vi "checkFinishPreparePassPlay.vi"(8 "error in (no error)":errorcluster, 10 "Game":refnum<class "Game.lvclass">, 11 "PreparePassPlay in":refnum<class "PreparePassPlay.lvclass">) -> (0 "error out":errorcluster, 2 "Boolean":bool, 3 "PreparePassPlay out":refnum<class "PreparePassPlay.lvclass">)   [LabVIEW 2018, in "PreparePassPlay.lvclass"]
uses:
  PreparePassPlay.lvclass
  Game_class/Game.lvclass
  Game_class/Game.lvclass/Game.ctl
  Referee_class/Referee.lvclass/Referee.ctl
  Events_class/Events.lvclass/Events.ctl
  Team_class/Team.lvclass/Team.ctl
  Referee_class/command_interpreted.ctl
  Game_class/Read OffensiveTeam.vi
  Team_class/Read OffensivePlay Finished.vi
  Game_class/Read EventsRef.vi
  Events_class/Read ball_out.vi
  Game_class/Read Referee.vi
  Referee_class/Read command_interpreted.vi
  Ally_class/Ally.lvclass
  C:/Users/anton/Desktop/roboime/Babulho do Testoni/SSL_AI/Team_class/Team.lvclass
  Referee_class/Referee.lvclass
  Events_class/Events.lvclass
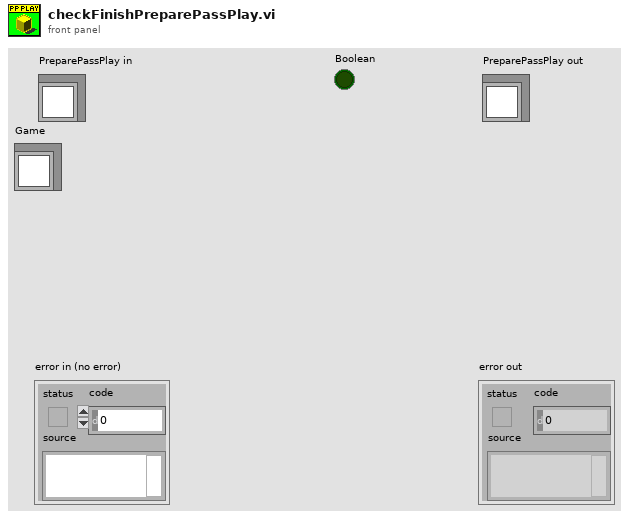
[diagram p1: front panel]
types:
  T1 = typedef "command_interpreted.ctl" = enum16{"Goal Ally", "Goal Enemy", "Ball Placement Enemy", "Ball Placement Ally", "Normal Half Time", "Extra Time  Break", "Extra Half Time", "None", "Post Game", "PKA Normal Start", "Prepare Kickoff Ally", "PKE Normal Start", "Prepare Kickoff Enemy", "Force Start", "Halt", "Timeout", "Prepare Penalty Ally", "Prepare Penalty Enemy", "PPA NormalStart", "PPE Normal Start", "Indirect Free Ally", "Direct Free Enemy", "Direct Free Ally", "Indirect Free Enemy", "Stop"}
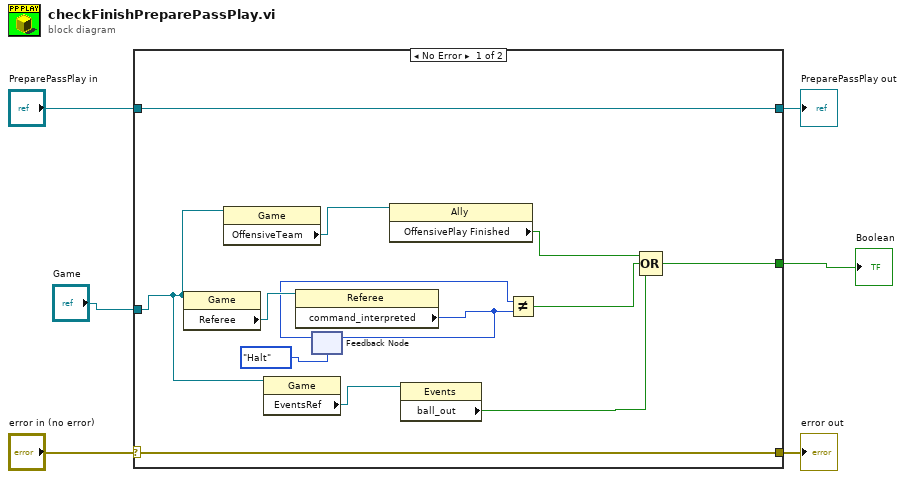
[diagram p0: block diagram]
diagram:
  n1 = case shown="No Error" "error in (no error)" {
    selector: "error in (no error)" -> [w18 w21]
    tunnel: [w18 w21] -> w5
    tunnel: [w19 w20] -> w3
    tunnel: "PreparePassPlay in" -> [w19 w20]
    tunnel: "Game" -> [w17 _]
    tunnel: [w7 _] -> w1
    frame No Error {
      n2 = property class="Game"(reference=w17) -> ("Referee"=w15:refnum<class "Referee.lvclass">)  [unwired: 1 in, 2 out]
      n3 = property class="Game"(reference=w17) -> ("OffensiveTeam"=w14:refnum<class "Ally.lvclass">)  [unwired: 1 in, 2 out]
      n4 = property class="Game"(reference=w17) -> ("EventsRef"=w16:refnum<class "Events.lvclass">)  [unwired: 1 in, 2 out]
      n5 = property class="Referee"(reference=w15) -> ("command_interpreted"=w11:T1)  [unwired: 1 in, 2 out]
      n6 = feedback-in #1(w11) -> ()
      n7 = feedback #1(command_interpreted."Halt" ("command_interpreted")) -> (w10:T1)
      n8 = property class="Ally"(reference=w14) -> ("OffensivePlay Finished"=w13:bool)  [unwired: 1 in, 2 out]
      n9 = property class="Events"(reference=w16) -> ("ball_out"=w12:bool)  [unwired: 1 in, 2 out]
      n10 = Not Equal?(x=w10, y=w11) -> (x != y?=w8:bool)
      n11 = Compound Arithmetic op=OR(w13, w8, w12) -> (w7:bool)
    }
    frame Error {
    }
  }
  "error out" <- w5
  "PreparePassPlay out" <- w3
  "Boolean" <- w1
